vi "Moving AVG&STDEV.vi"(3 "Clear the Array:  True \n Add New Value:  False":bool, 4 "New Element for Moving Window":dbl, 5 "Initial Array":dbl[](array[numeric])) -> (0 "Standard Dev":dbl, 1 "Arithmetic Mean":dbl, 2 "Moving Window Array":dbl[](array[numeric]))   [LabVIEW 2017]
uses:
  Instance           2 24Saved   Moving AVG&STDEV .vi
  Instance           1 24Saved   Moving AVG&STDEV .vi
panel:
  # "Moving Window Average and Standard Deviation\n- W. Vance Payne, BFRL, NIST\n- modified by Minsung Kim, 11/18/2005"
  # "* Set to TRUE to clear an existing array; \n    otherwise set to FALSE to add new elements."
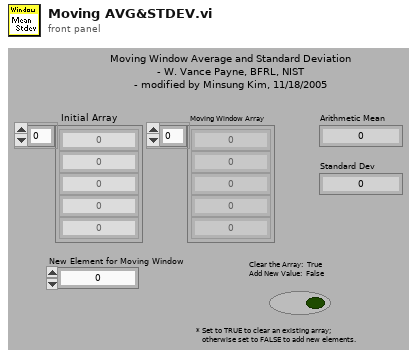
[diagram p1: front panel]
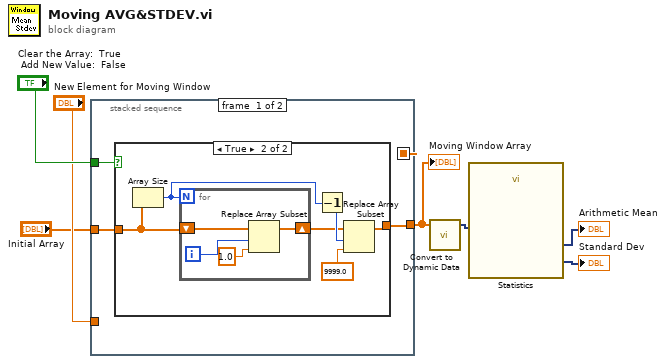
[diagram p0: block diagram]
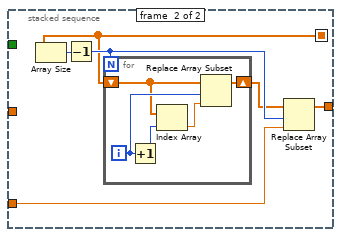
[diagram p3: hidden frame]
diagram:
  n1 = stacked-sequence {
    seq-local: [w9 _] -> [_ w23]
    tunnel: "Clear the Array:  True \n Add New Value:  False" -> [w10 _]
    tunnel: "New Element for Moving Window" -> [_ w26]
    tunnel: [_ w25] -> w5
    tunnel: "Initial Array" -> [w8 _]
    frame #0 {
      n2 = case shown="True" w10 {
        tunnel: [w11 w14] -> w9
        tunnel: w8 -> [w11 w12]
        frame False {
        }
        frame True {
          n3 = Array Size(array=w12) -> (size(s)=w15:i32)
          n4 = for {
            N: w15 -> [_]
            shift-right: [w18] -> w13
            shift-left: w12 -> [w19]
            i -> [w21]
            n5 = Replace Array Subset(array=w19, new element=1.0 ("new element/subarray"), index=w21) -> (w18:dbl[])
          }
          n6 = Decrement(x=w15) -> (x-1=w16:i32)
          n7 = Replace Array Subset(array=w13, new element=9999.0 ("new element/subarray"), index=w16) -> (w14:dbl[])
        }
      }
    }
    frame #1 {
      n8 = Array Size(array=w23) -> (size(s)=w27:i32)
      n9 = Decrement(x=w27) -> (x-1=w24:i32)
      n10 = for {
        N: w24 -> [_]
        shift-right: [w28] -> w22
        shift-left: w23 -> [w29]
        i -> [w31]
        n11 = Increment(x=w31) -> (x+1=w32:i32)
        n12 = Index Array(array=w29, index=w32) -> (element=w30:dbl)
        n13 = Replace Array Subset(array=w29, new element=w30, index=w31) -> (w28:dbl[])
      }
      n14 = Replace Array Subset(array=w22, new element=w26, index=w24) -> (w25:dbl[])
    }
  }
  "Moving Window Array" <- w5
  n15 = call "Convert to Dynamic Data"("Array"=w5) -> ("Dynamic Data Type"=w4:dynamicdata)  [unwired: 3 out]
  n16 = call "Statistics"("Signals"=w4) -> ("Standard Dev"=→"Standard Dev":dynamicdata, "Arithmetic Mean"=→"Arithmetic Mean":dynamicdata)  [unwired: 1 in, 24 out]
